vi "Upload program time.vi"(7 "Address":dbl=1.0, 8 "error in (no error)":errorcluster, 9 "Segment":dbl=6.0, 10 "Time":dbl=10.0, 11 "VISA resource name (IN)":refnum<visa-resource-name>) -> (0 "error out":errorcluster, 3 "VISA resource name (OUT)":refnum<visa-resource-name>)   [LabVIEW 2010, in "Yudian AI508.lvlib"]
doc: "Use this template to build a VI to use as a subVI."
uses:
  <instrlib>/Yudian AI508/Yudian AI508.lvlib
panel:
  out "Recieved Raw Data":string
  out "Recevied Temp.  data":dbl
  out "Data buffer":string
  out "Digital shift":i32
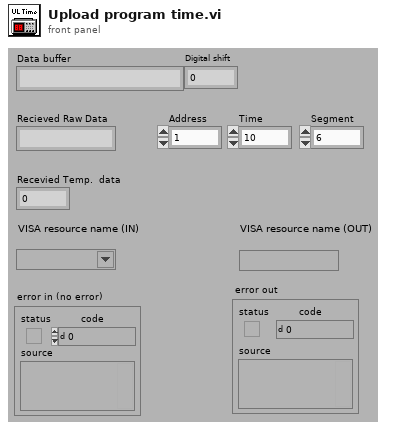
[diagram p1: front panel]
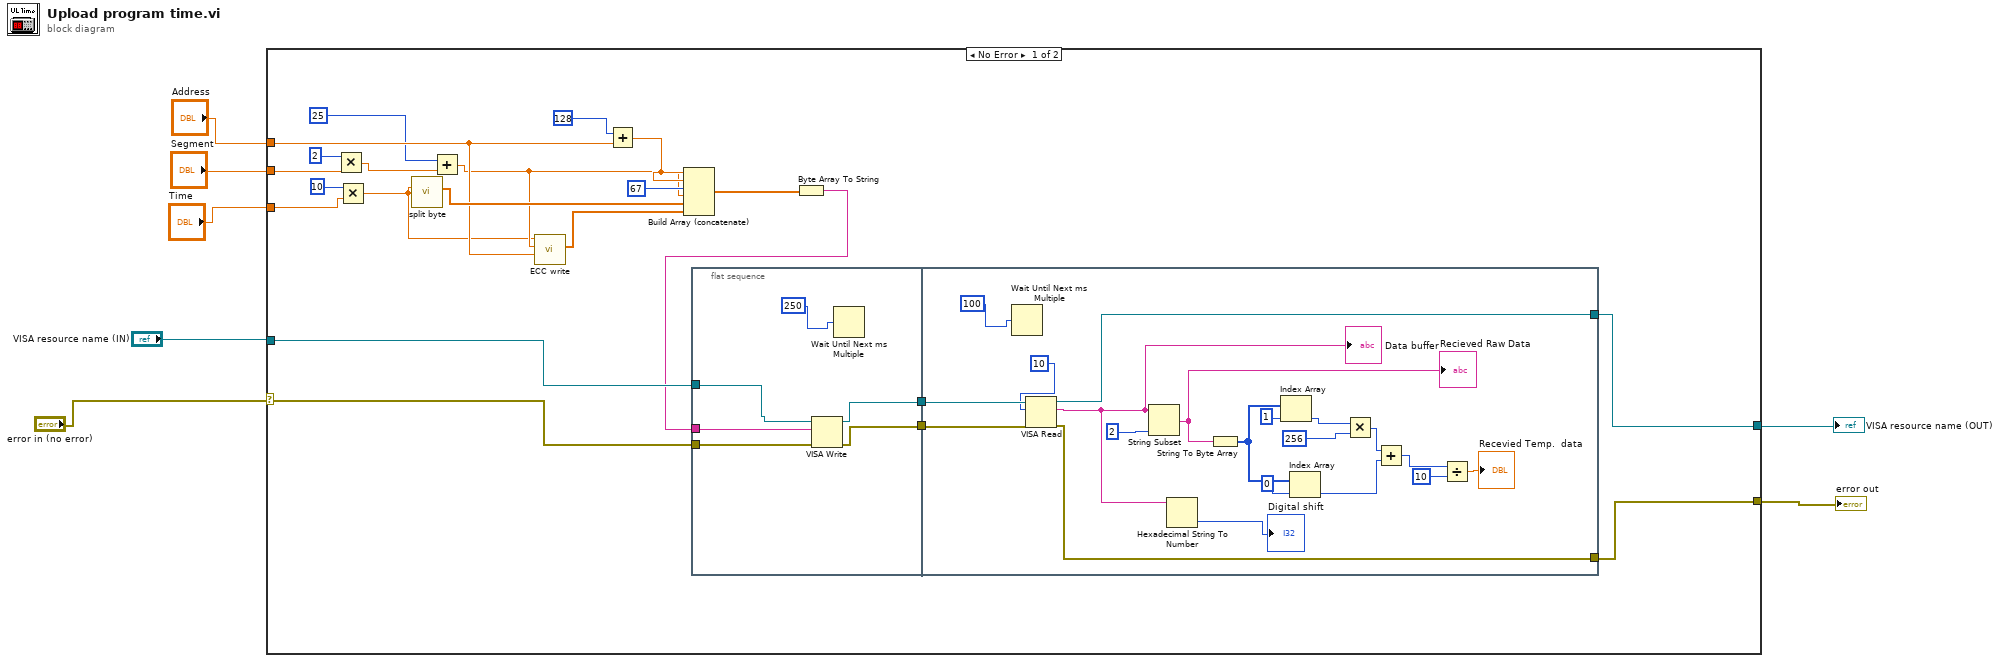
[diagram p0: block diagram]
diagram:
  n1 = case shown="No Error" "error in (no error)" {
    selector: "error in (no error)" -> [w24 w57]
    tunnel: [w26 w57] -> w7
    tunnel: [w27 w56] -> w6
    tunnel: "VISA resource name (IN)" -> [w25 w56]
    tunnel: "Address" -> [w19 _]
    tunnel: "Segment" -> [w15 _]
    tunnel: "Time" -> [w8 _]
    frame No Error {
      n2 = Multiply(x=2, y=w15) -> (x*y=w13:dbl)
      n3 = Multiply(x=10, y=w8) -> (x*y=w10:dbl)
      n4 = call <instrlib>:"split byte.vi"("Value"=w10) -> ("Array"=w20:dbl[])  [unwired: 10 in]
      n5 = Add(x=25, y=w13) -> (x+y=w16:dbl)
      n6 = call <instrlib>:"ECC write.vi"("Address"=w19, "Parameter code"=w16, "Value"=w10) -> ("Data array"=w18:dbl[])  [unwired: 8 in]
      n7 = Add(x=128, y=w19) -> (x+y=w23:dbl)
      n8 = Build Array (concatenate)(w23, w23, 67, w16, w20, w18) -> (w12:dbl[])
      n9 = flat-sequence {
        tunnel: w24 -> [w35]
        tunnel: w25 -> [w32]
        tunnel: [w34] -> w29
        tunnel: [w33] -> w28
        tunnel: w11 -> [w30]
        tunnel: w29 -> [w41]
        tunnel: w28 -> [w40]
        tunnel: [w38] -> w27
        tunnel: [w37] -> w26
        frame #0 {
          n10 = VISA Write(VISA resource name=w32, write buffer=w30, error in (no error)=w35) -> (VISA resource name out=w33:refnum<visa-resource-name>, error out=w34:errorcluster)  [unwired: 1 out]
          n11 = Wait Until Next ms Multiple(millisecond multiple=250) -> ()  [unwired: 1 out]
        }
        frame #1 {
          n12 = Wait Until Next ms Multiple(millisecond multiple=100) -> ()  [unwired: 1 out]
          n13 = VISA Read(VISA resource name=w40, byte count=u32 10 ("字节总数"), error in (no error)=w41) -> (VISA resource name out=w38:refnum<visa-resource-name>, read buffer=w43:string, error out=w37:errorcluster)  [unwired: 1 out]
          "Data buffer" <- w43
          n14 = String Subset(string=w43, length (rest)=2 ("length (rest)")) -> (substring=w53:string)  [unwired: 1 out]
          "Recieved Raw Data" <- w53
          n15 = Hexadecimal String To Number(string=w43) -> (number=→"Digital shift":u32)  [unwired: 3 out]
          n16 = String To Byte Array(string=w53) -> (unsigned byte array=w51:u8[])
          n17 = Index Array(array=w51, index=1) -> (element=w50:u8)
          n18 = Index Array(array=w51, index=0) -> (element=w47:u8)
          n19 = Multiply(x=w50, y=u16 256) -> (x*y=w48:u16)
          n20 = Add(x=w48, y=w47) -> (x+y=w46:u16)
          n21 = Divide(x=w46, y=u16 10) -> (x/y=→"Recevied Temp.  data":dbl)
        }
      }
      n22 = Byte Array To String(unsigned byte array=w12) -> (string=w11:string)
    }
    frame Error {
    }
  }
  "error out" <- w7
  "VISA resource name (OUT)" <- w6
